vi "Raster_2DOutput_wCounter_82_FLIM_Trigger.vi"(2 "Save File path":path, 3 "Save?":bool=TRUE, 6 "error in":errorcluster, 7 "Update Rate (Hz)":dbl=100.0, 8 "Y Parameters":T1={"Number of Y Steps"=200, "Max Y (V)"=2.0, "Min Y (V)"=-2.0}, 9 "X Parameters":T2={"Number of X Steps"=200, "Max X (V)"=2.0, "Min X (V)"=-2.0}) -> (0 "error out":errorcluster, 1 "Intensity Graph":dbl[][](graph))   [LabVIEW 2011]
uses:
  <vilib>/DAQmx/write.llb/DAQmx Write (Analog 2D DBL NChan NSamp).vi
  <vilib>/DAQmx/read.llb/DAQmx Read (Counter 1D U32 1Chan NSamp).vi
  <vilib>/DAQmx/create/channels.llb/DAQmx Create Channel (CI-Count Edges).vi
  <vilib>/DAQmx/create/channels.llb/DAQmx Create Channel (AO-Voltage-Basic).vi
  <vilib>/DAQmx/configure/timing.llb/DAQmx Timing (Sample Clock).vi
  <vilib>/DAQmx/configure/trigger.llb/DAQmx Start Trigger (Digital Edge).vi
  <vilib>/DAQmx/miscellaneous.llb/DAQmx Fill In Error Info.vi
  Program Files/National Instruments/LabVIEW 2011/resource/objmgr/daqmx.rc
panel:
  out "TotalSampPerChanAcquired":dbl
  out "Output:":dbl[][](graph)
  in  "stop":bool
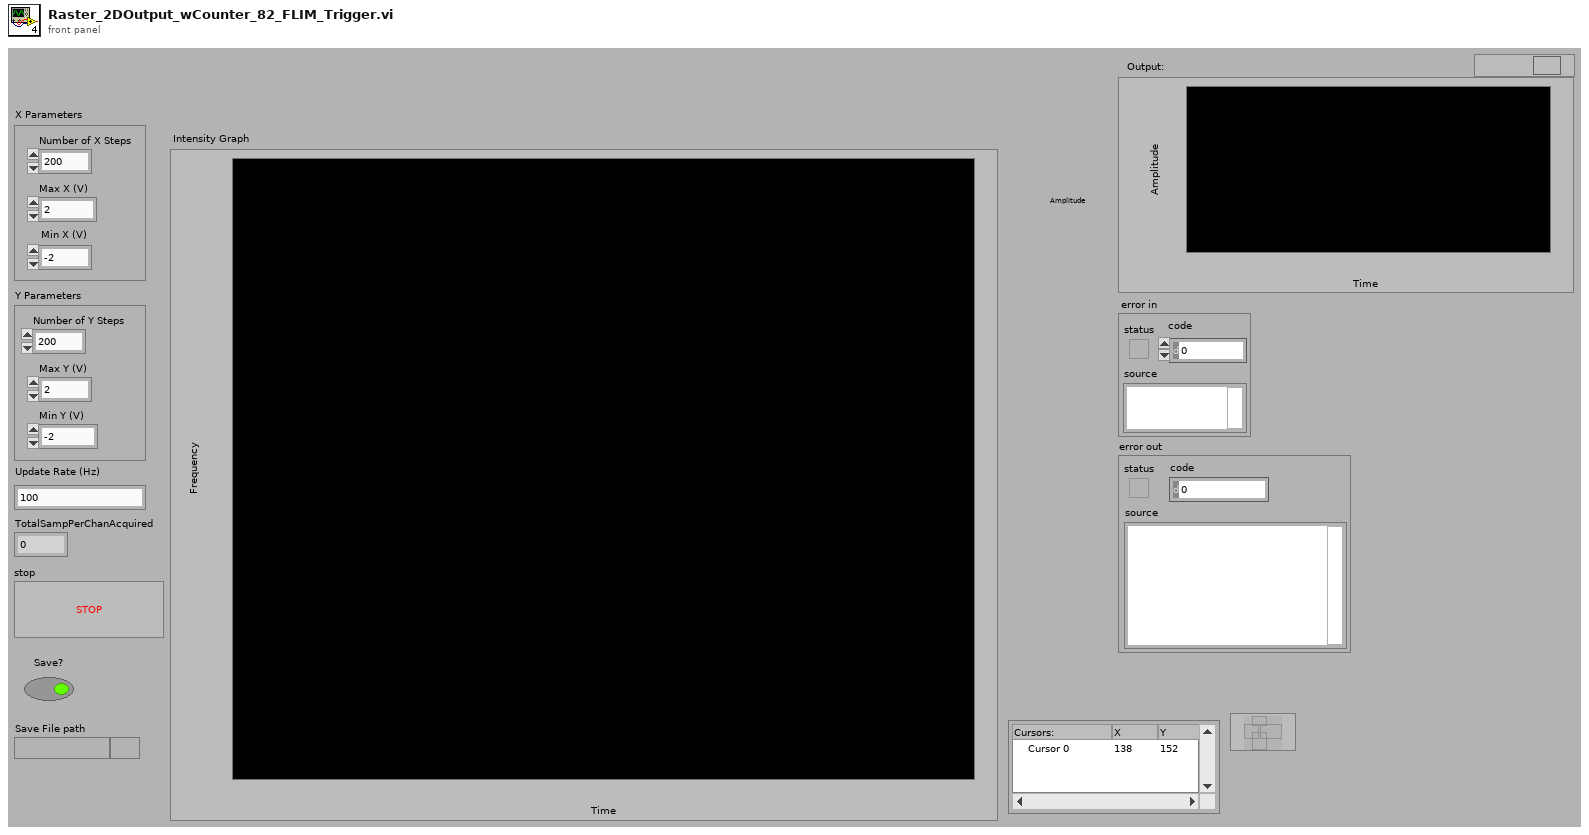
[diagram p1: front panel]
types:
  T1 = cluster{"Number of Y Steps":i32, "Max Y (V)":dbl, "Min Y (V)":dbl}
  T2 = cluster{"Number of X Steps":i32, "Max X (V)":dbl, "Min X (V)":dbl}
  T3 = typedef "imagedata.ctl" = cluster{"image type":i32, "image depth":i32, "image":u8[], "mask":u8[], "colors":u32[], "Rectangle":cluster{"left":i16, "top":i16, "right":i16, "bottom":i16}}
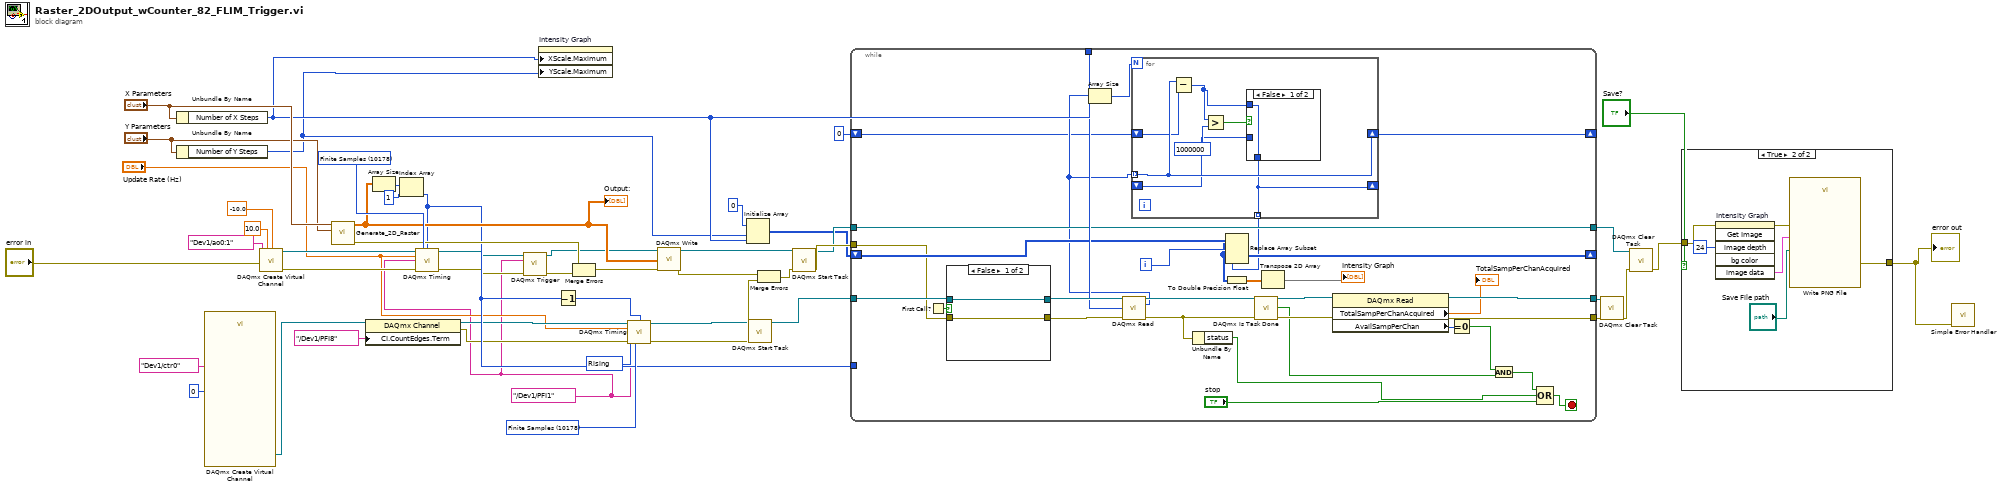
[diagram p0: block diagram]
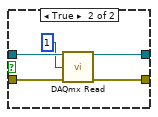
[diagram p4: hidden frame]
diagram:
  w7 = 10280 items=["Rising"=10280, "Falling"=10171] ("active edge")
  w1 = tag "/Dev1/PFI1" ("source")
  w43 = 10178 items=["Finite Samples"=10178, "Continuous Samples"=10123, "Hardware Timed Single Point"=12522] ("sample mode")
  w44 = 10178 items=["Finite Samples"=10178, "Continuous Samples"=10123, "Hardware Timed Single Point"=12522] ("sample mode")
  n1 = Unbundle By Name("X Parameters") -> ("Number of X Steps"=w12:i32)
  n2 = Unbundle By Name("Y Parameters") -> ("Number of Y Steps"=w11:i32)
  n3 = call-poly <vilib>:"DAQmx Create Virtual Channel.vi"("initial count"=u32 0, "counter"=tag "Dev1/ctr0") -> ("task out"=w20:refnum<k21>)  [unwired: 6 in, 7 out]
  n4 = call-poly <vilib>:"DAQmx Create Virtual Channel.vi"("maximum value"=10.0, "minimum value"=-10.0, "physical channels"=tag "Dev1/ao0:1", "error in"="error in") -> ("task out"=w51:refnum<k21>, "error out"=w50:errorcluster)  [unwired: 5 in, 5 out]
  n5 = call "Generate_2D_Raster.vi"("Y Parameters"="Y Parameters", "X Parameters"="X Parameters") -> ("error IO"=w35:errorcluster, "Array"=w30:dbl[][])  [unwired: 1 in, 7 out]
  "Output:" <- w30
  n6 = property class="DAQmx Channel"(reference=w20, "CI.CountEdges.Term"=tag "/Dev1/PFI8") -> (reference out=w19:refnum<k21>, error out=w16:errorcluster)  [unwired: 1 in]
  n7 = Array Size(array=w30) -> (size(s)=w29:i32[])
  n8 = Index Array(array=w29, index=1) -> (element=w27:i32)
  n9 = call-poly <vilib>:"DAQmx Timing.vi"("task/channels in"=w51, "sample mode"=w44, "samples per channel"=w27, "rate"="Update Rate (Hz)", "source"=w1, "error in"=w50) -> ("task out"=w6:refnum<k21>, "error out"=w5:errorcluster)  [unwired: 1 in, 7 out]
  n10 = call-poly <vilib>:"DAQmx Trigger.vi"("task/channels in"=w6, "source"=w1, "error in"=w5) -> ("task out"=w2:refnum<k21>, "error out"=w3:errorcluster)  [unwired: 11 in]
  n11 = property on="Intensity Graph" class="IntGraph (strict)"("XScale.Maximum"=w12, "YScale.Maximum"=w11) -> ()  [unwired: 2 in, 2 out]
  n12 = Decrement(x=w27) -> (x-1=w24:i32)
  n13 = Merge Errors(w35, w3) -> (w4:errorcluster)
  n14 = call-poly <vilib>:"DAQmx Timing.vi"("task/channels in"=w19, "sample mode"=w43, "samples per channel"=w24, "rate"="Update Rate (Hz)", "source"=w1, "active edge"=w7, "error in"=w16) -> ("task out"=w9:refnum<k21>, "error out"=w8:errorcluster)  [unwired: 7 out]
  n15 = call-poly <vilib>:"DAQmx Write.vi"("task/channels in"=w2, "data"=w30, "error in"=w4) -> ("task out"=w48:refnum<k21>, "error out"=w37:errorcluster)  [unwired: 1 in, 10 out]
  n16 = Initialize Array(u32 0, w11, w12) -> (w31:u32[][])
  n17 = call <vilib>:"DAQmx Start Task.vi"("task/channels in"=w9, "error in"=w8) -> ("task out"=w45:refnum<k21>, "error out"=w36:errorcluster)  [unwired: 12 out]
  n18 = Merge Errors(w37, w36) -> (w38:errorcluster)
  n19 = call <vilib>:"DAQmx Start Task.vi"("task/channels in"=w48, "error in"=w38) -> ("task out"=w46:refnum<k21>, "error out"=w47:errorcluster)  [unwired: 12 out]
  n20 = while {
    tunnel: w46 -> [w72]
    tunnel: w47 -> [w73]
    tunnel: w45 -> [w81]
    tunnel: [w72] -> w42
    tunnel: w12 -> [w77]
    shift-right: [w74] -> _
    shift-left: w31 -> [w76]
    tunnel: w27 -> [_]
    tunnel: [w68] -> w26
    tunnel: [w69] -> w25
    shift-right: [w54] -> _
    shift-left: u32 0 ("Numeric") -> [w53]
    i -> [w75]
    stop <- w82 stop-if-true
    n21 = First Call?() -> (First Call?: T/F=w78:bool)
    n22 = case shown="False" w78 {
      tunnel: w81 -> [w93 w98]
      tunnel: [w93 w97] -> w80
      tunnel: [w92 w96] -> w79
      tunnel: w73 -> [w92 w95]
      frame False {
      }
      frame True {
        n23 = call-poly <vilib>:"DAQmx Read.vi"("task/channels in"=w98, "number of samples per channel"=1, "error in"=w95) -> ("task out"=w97:refnum<k21>, "error out"=w96:errorcluster)  [unwired: 11 out]
      }
    }
    n24 = call-poly <vilib>:"DAQmx Read.vi"("task/channels in"=w80, "number of samples per channel"=w77, "error in"=w79) -> ("task out"=w70:refnum<k21>, "data"=w56:u32[], "error out"=w61:errorcluster)  [unwired: 1 in, 9 out]
    n25 = Array Size(array=w56) -> (size(s)=w57:i32)
    n26 = for {
      N: w57 -> [_]
      tunnel: w56 -> [w89] mode=indexing
      shift-right: [w89] -> w54
      shift-left: w53 -> [w88]
      tunnel: [w84] -> w55 mode=indexing
      shift-right: [w84] -> _
      shift-left: _ -> [w83]
      n27 = Subtract(x=w89, y=w88) -> (x-y=w85:u32)
      n28 = Greater?(x=w85, y=u32 1000000) -> (0:w86:bool)
      n29 = case shown="False" w86 {
        tunnel: w85 -> [w90 _]
        tunnel: [w90 w91] -> w84
        tunnel: w83 -> [_ w91]
        frame False {
        }
        frame True {
        }
      }
    }
    n30 = Unbundle By Name(w61) -> ("status"=w59:bool)
    n31 = Replace Array Subset(array=w76, new element=w55, index (row)=w75) -> (w74:u32[][])  [unwired: 1 in]
    n32 = To Double Precision Float(number=w74) -> (double precision float=w71:dbl[][])
    n33 = call <vilib>:"DAQmx Is Task Done.vi"("task/channels in"=w70, "error in"=w61) -> ("task out"=w67:refnum<k21>, "task done?"=w64:bool, "error out"=w66:errorcluster)  [unwired: 11 out]
    n34 = Transpose 2D Array(2D array=w71) -> (transposed array=→"Intensity Graph":dbl[][])
    n35 = property class="DAQmx Read"(reference=w67, error in=w66) -> (reference out=w69:refnum<k21>, error out=w68:errorcluster, "TotalSampPerChanAcquired"=→"TotalSampPerChanAcquired":dbl, "AvailSampPerChan"=w63:u32)
    n36 = Equal To 0?(x=w63) -> (x = 0?=w62:bool)
    n37 = And(x=w62, y=w64) -> (x .and. y?=w58:bool)
    n38 = Compound Arithmetic op=OR(w58, w59, "stop") -> (w82:bool)
  }
  n39 = call <vilib>:"DAQmx Clear Task.vi"("task in"=w25, "error in"=w26) -> ("error out"=w39:errorcluster)  [unwired: 13 out]
  n40 = call <vilib>:"DAQmx Clear Task.vi"("task in"=w42, "error in"=w39) -> ("error out"=w23:errorcluster)  [unwired: 13 out]
  n41 = case shown="True" "Save?" {
    tunnel: w23 -> [w99 w103]
    tunnel: [w99 w105] -> w10
    frame False {
    }
    frame True {
      n42 = invoke on="Intensity Graph" class="IntGraph (strict)" method="Get Image"(error in=w103, "image depth"=24 ("Image Depth")) -> (error out=w102:errorcluster, "image data"=w101:T3)  [unwired: 4 in, 4 out]
      n43 = call <vilib>:"Write PNG File.vi"("error in (no error)"=w102, "image data"=w101, "path to PNG file"="Save File path") -> ("error out"=w105:errorcluster)  [unwired: 7 in, 1 out]
    }
  }
  "error out" <- w10
  n44 = call <vilib>:"Simple Error Handler.vi"("error in (no error)"=w10) -> ()  [unwired: 4 in, 5 out]
